vi "AlarmReport.vi"(5 "PalletError":i32, 6 "RooCauseIn":string, 7 "Emun":T1=enum."WriteOPID", 8 "VILinkerror In":errorcluster, 9 "OPID":string, 10 "error In":errorcluster, 11 "ErrorTableIn":refnum<vi>) -> (0 "error out":errorcluster)   [LabVIEW 2019]
uses:
  Ctrl/AlarmReportCtrl.ctl
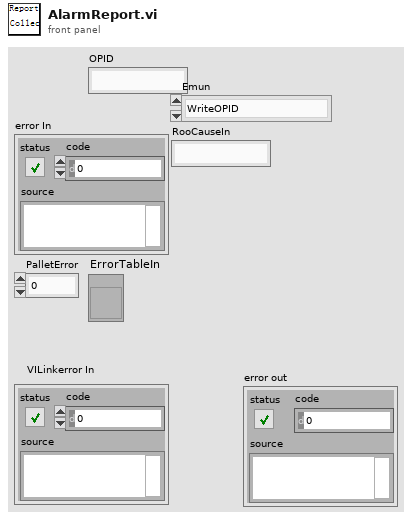
[diagram p1: front panel]
types:
  T1 = typedef "AlarmReportCtrl.ctl" = enum16{"Initial", "AddError", "WriteAlarmResetTime", "WriteOPID", "Load", "Save", "WriteRootCause"}
  T2 = enum16{"open", "replace", "create", "open or create", "replace or create", "replace or create with confirmation"}
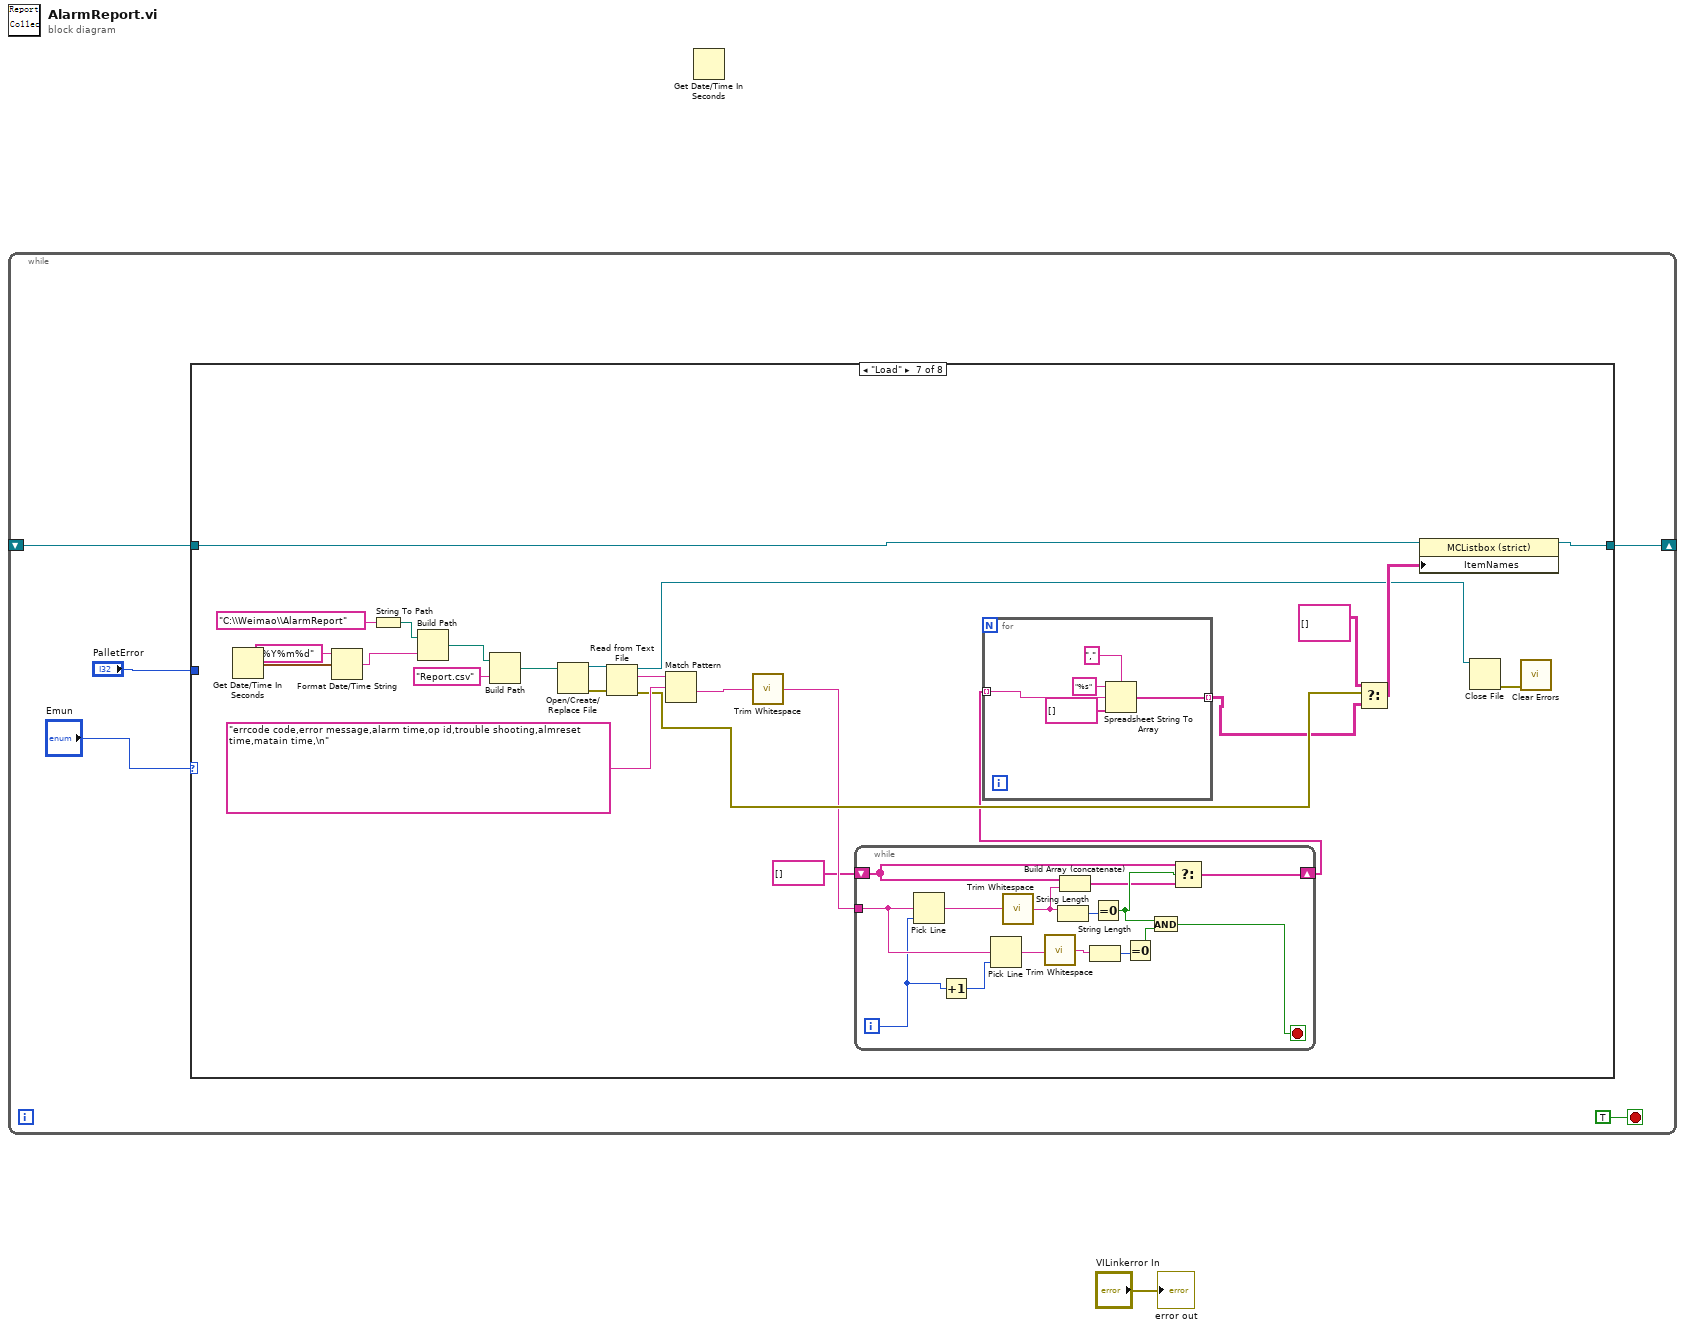
[diagram p0: block diagram]
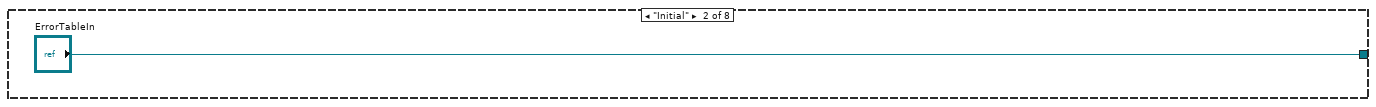
[diagram p3: hidden frame]
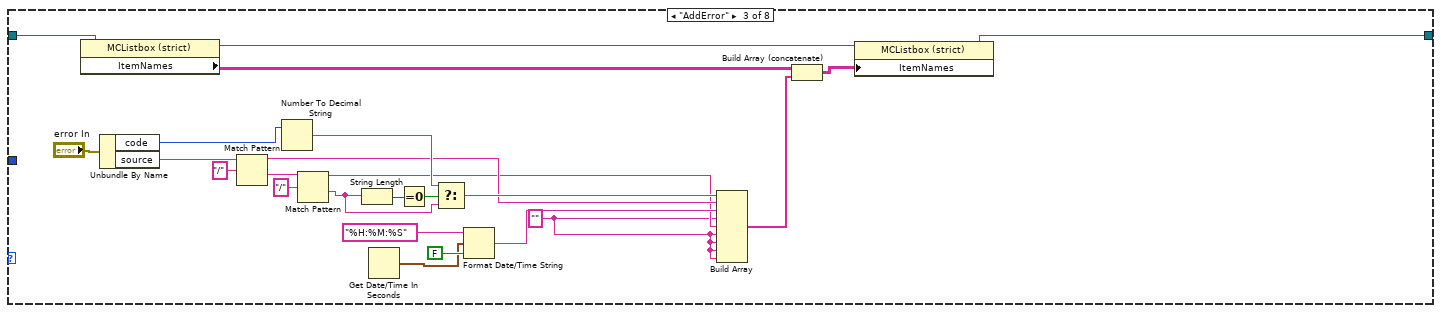
[diagram p4: hidden frame]
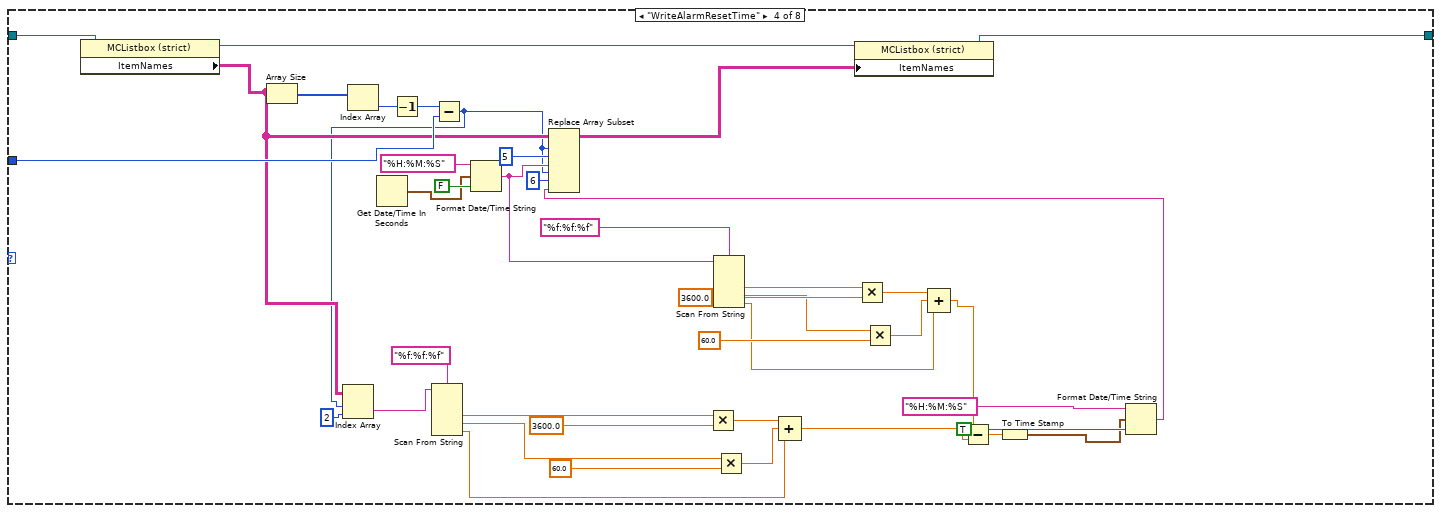
[diagram p5: hidden frame]
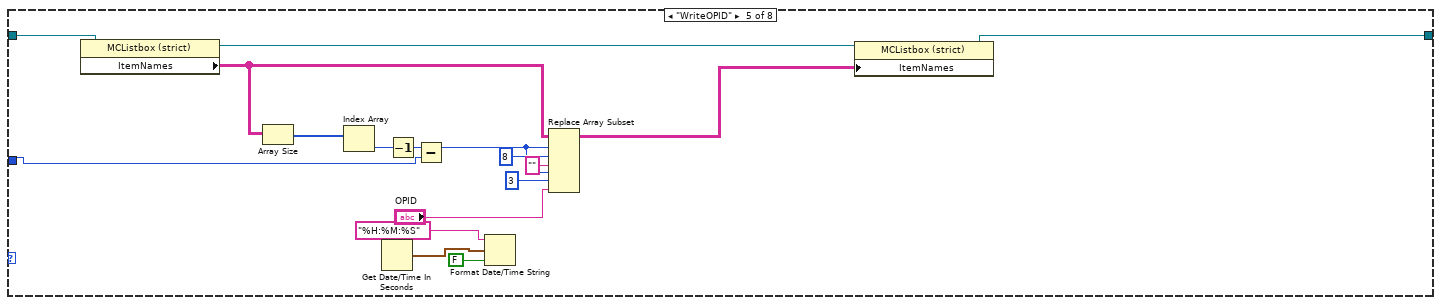
[diagram p6: hidden frame]
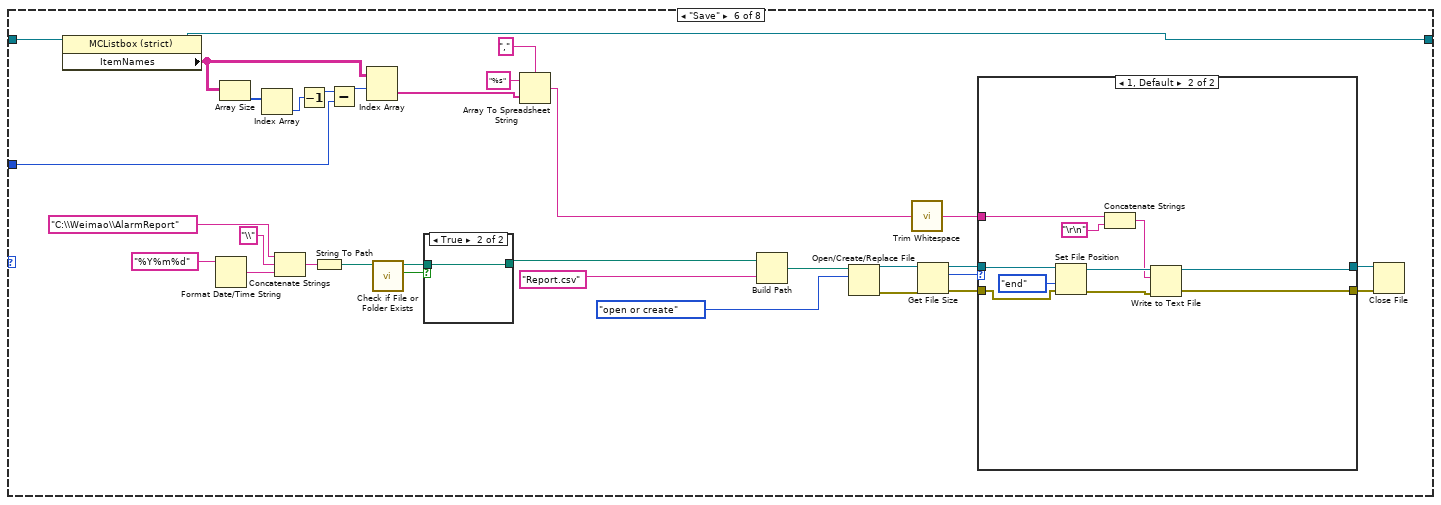
[diagram p7: hidden frame]
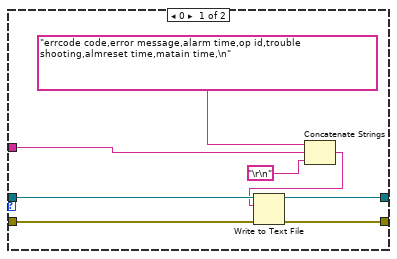
[diagram p8: hidden frame]
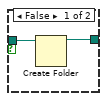
[diagram p9: hidden frame]
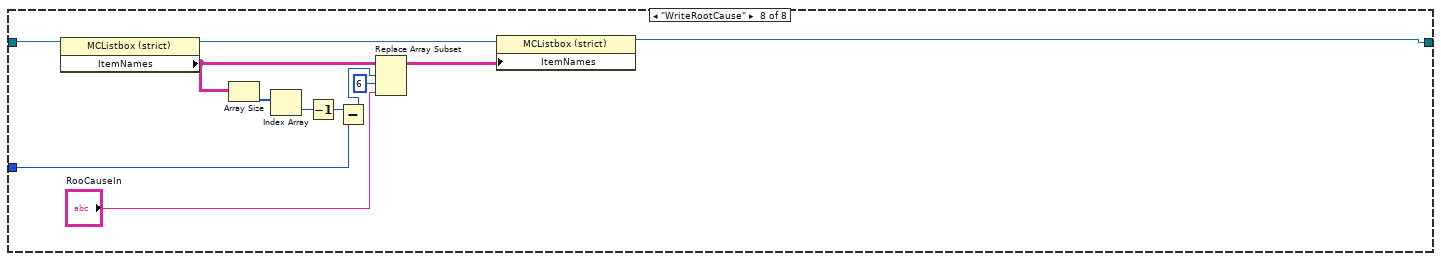
[diagram p10: hidden frame]
diagram:
  n1 = while {
    shift-right: [w4] -> _
    shift-left: _ -> [w3]
    stop <- TRUE stop-if-true
    n2 = case shown="\"Load\"" "Emun" {
      tunnel: [w7 "ErrorTableIn" w12 w71 w88 w121 w166 w191] -> w4
      tunnel: w3 -> [w7 _ w32 w73 w90 w122 w167 w199]
      tunnel: "PalletError" -> [_ _ _ w61 w76 w91 _ w188]
      frame Default {
      }
      frame "Initial" {
      }
      frame "AddError" {
        w15 = "" ("element")
        n3 = property class="MCListbox (strict)"(reference=w32) -> (reference out=w14:refnum<vi>, "ItemNames"=w30:string[][])  [unwired: 1 in, 1 out]
        n4 = Unbundle By Name("error In") -> ("code"=w23:i32, "source"=w29:string)
        n5 = Match Pattern(string=w29, regular expression="/") -> (before substring=w19:string, after substring=w27:string)  [unwired: 1 in, 2 out]
        n6 = Number To Decimal String(number=w23) -> (decimal integer string=w22:string)  [unwired: 1 in]
        n7 = Match Pattern(string=w27, regular expression="/") -> (before substring=w16:string, after substring=w21:string)  [unwired: 1 in, 2 out]
        n8 = String Length(string=w21) -> (length=w25:i32)
        n9 = Get Date/Time In Seconds() -> (seconds since 1Jan1904=w10:timestamp)
        n10 = Equal To 0?(x=w25) -> (x = 0?=w24:bool)
        n11 = Select(t=w22, s=w24, f=w21) -> (s? t:f=w20:string)
        n12 = Format Date/Time String(time format string (%c)="%H:%M:%S", seconds (now)=w10, UTC format=FALSE) -> (date/time string=w17:string)
        n13 = Build Array(w20, w19, w17, w15, w16, w15, w15, w15, w15) -> (w9:string[])
        n14 = Build Array (concatenate)(w30, w9) -> (w13:string[][])
        n15 = property class="MCListbox (strict)"(reference=w14, "ItemNames"=w13) -> (reference out=w12:refnum<vi>)  [unwired: 1 in, 1 out]
      }
      frame "WriteAlarmResetTime" {
        n16 = property class="MCListbox (strict)"(reference=w73) -> (reference out=w72:refnum<vi>, "ItemNames"=w57:string[][])  [unwired: 1 in, 1 out]
        n17 = Array Size(array=w57) -> (size(s)=w69:i32[])
        n18 = Index Array(array=w69) -> (element=w68:i32)  [unwired: 1 in]
        n19 = Get Date/Time In Seconds() -> (seconds since 1Jan1904=w62:timestamp)
        n20 = Decrement(x=w68) -> (x-1=w65:i32)
        n21 = Subtract(x=w65, y=w61) -> (x-y=w33:i32)
        n22 = Index Array(array=w57, index (row)=w33, index (col)=2 ("disabled index (col)")) -> (element=w41:string)
        n23 = Scan From String(format string="%f:%f:%f", input string=w41) -> (output 1=w43:dbl, output 2=w45:dbl, output 3=w49:dbl)  [unwired: 5 in, 3 out]
        n24 = Format Date/Time String(time format string (%c)="%H:%M:%S", seconds (now)=w62, UTC format=FALSE) -> (date/time string=w59:string)
        n25 = Multiply(x=w43, y=3600.0) -> (x*y=w47:dbl)
        n26 = Scan From String(format string="%f:%f:%f", input string=w59) -> (output 1=w58:dbl, output 2=w54:dbl, output 3=w50:dbl)  [unwired: 5 in, 3 out]
        n27 = Multiply(x=w45, y=60.0) -> (x*y=w48:dbl)
        n28 = Compound Arithmetic op=ADD(w47, w48, w49) -> (w35:dbl)
        n29 = Multiply(x=w58, y=3600.0) -> (x*y=w52:dbl)
        n30 = Multiply(x=w54, y=60.0) -> (x*y=w51:dbl)
        n31 = Compound Arithmetic op=ADD(w52, w51, w50) -> (w34:dbl)
        n32 = Subtract(x=w34, y=w35) -> (x-y=w40:dbl)
        n33 = To Time Stamp(1:w40) -> (0:w37:timestamp)
        n34 = Format Date/Time String(time format string (%c)="%H:%M:%S", seconds (now)=w37, UTC format=TRUE) -> (date/time string=w36:string)
        n35 = Replace Array Subset(array=w57, new element #1=w59, index (row) #1=w33, index (col) #1=5 ("disabled index (col)"), new element #2=w36, index (row) #2=w33, index (col) #2=6 ("disabled index (col)")) -> (w70:string[][])
        n36 = property class="MCListbox (strict)"(reference=w72, "ItemNames"=w70) -> (reference out=w71:refnum<vi>)  [unwired: 1 in, 1 out]
      }
      frame "WriteOPID" {
        n37 = property class="MCListbox (strict)"(reference=w90) -> (reference out=w89:refnum<vi>, "ItemNames"=w83:string[][])  [unwired: 1 in, 1 out]
        n38 = Array Size(array=w83) -> (size(s)=w86:i32[])
        n39 = Index Array(array=w86) -> (element=w85:i32)  [unwired: 1 in]
        n40 = Get Date/Time In Seconds() -> (seconds since 1Jan1904=w78:timestamp)
        n41 = Decrement(x=w85) -> (x-1=w81:i32)
        n42 = Subtract(x=w81, y=w76) -> (x-y=w77:i32)
        n43 = Format Date/Time String(time format string (%c)="%H:%M:%S", seconds (now)=w78, UTC format=FALSE) -> ()  [unwired: 1 out]
        n44 = Replace Array Subset(array=w83, new element #1="" ("new element/subarray"), index (row) #1=w77, index (col) #1=8 ("disabled index (col)"), new element #2="OPID", index (row) #2=w77, index (col) #2=3 ("disabled index (col)")) -> (w87:string[][])
        n45 = property class="MCListbox (strict)"(reference=w89, "ItemNames"=w87) -> (reference out=w88:refnum<vi>)  [unwired: 1 in, 1 out]
      }
      frame "Save" {
        n46 = property class="MCListbox (strict)"(reference=w122) -> (reference out=w121:refnum<vi>, "ItemNames"=w105:string[][])  [unwired: 1 in, 1 out]
        n47 = Format Date/Time String(time format string (%c)="%Y%m%d") -> (date/time string=w118:string)  [unwired: 2 out]
        n48 = Array Size(array=w105) -> (size(s)=w104:i32[])
        n49 = Index Array(array=w104) -> (element=w103:i32)  [unwired: 1 in]
        n50 = Concatenate Strings("C:\\Weimao\\AlarmReport" ("LogFolder"), "\\" ("string"), w118) -> (w117:string)
        n51 = Decrement(x=w103) -> (x-1=w92:i32)
        n52 = String To Path(string=w117) -> (path=w115:path)
        n53 = Subtract(x=w92, y=w91) -> (x-y=w93:i32)
        n54 = Index Array(array=w105, index (row)=w93) -> (element=w102:string[])  [unwired: 1 in]
        n55 = call <vilib>:"Check if File or Folder Exists.vi"("path"=w115) -> ("file or folder exists?"=w113:bool, "dup path"=w114:path)  [unwired: 8 in, 1 out]
        n56 = case shown="True" w113 {
          tunnel: w114 -> [w142 w143]
          tunnel: [w141 w143] -> w112
          frame False {
            n57 = Create Folder(path (use dialog)=w142) -> (created path=w141:path)  [unwired: 2 in, 2 out]
          }
          frame True {
          }
        }
        n58 = Array To Spreadsheet String(delimiter (Tab)=",", array=w102, 3:"%s" ("format string")) -> (spreadsheet string=w99:string)
        n59 = Build Path(base path=w112, name or relative path="Report.csv") -> (appended path=w110:path)
        n60 = Open/Create/Replace File(file path (use dialog)=w110, operation (0:open)=T2."open or create") -> (refnum out=w108:refnum<file>, error out=w107:errorcluster)  [unwired: 4 in, 1 out]
        n61 = call <vilib>:"Trim Whitespace.vi"("string"=w99) -> ("trimmed string"=w94:string)  [unwired: 1 in]
        n62 = Get File Size(file=w108, error in=w107) -> (refnum out=w98:refnum<file>, size (in bytes)=w106:i64, 0:w97:errorcluster)
        n63 = case shown="1, Default" w106 {
          tunnel: w94 -> [w129 w135]
          tunnel: w98 -> [w128 w140]
          tunnel: w97 -> [w127 w138]
          tunnel: [w126 w134] -> w95
          tunnel: [w125 w133] -> w96
          frame 0 {
            n64 = Concatenate Strings("errcode code,error message,alarm time,op id,trouble shooting,almreset time,matain time,\n", w129, "\r\n") -> (w123:string)
            n65 = Write to Text File(file (use dialog)=w128, text=w123, error in=w127) -> (refnum out=w126:refnum<file>, error out=w125:errorcluster)  [unwired: 1 in, 1 out]
          }
          frame 1, Default {
            n66 = Set File Position(refnum=w140, from (0:start)=enum16{"start", "end", "current"}."end", error in=w138) -> (refnum out=w137:refnum<file>, error out=w136:errorcluster)  [unwired: 1 in]
            n67 = Concatenate Strings(w135, "\r\n") -> (w132:string)
            n68 = Write to Text File(file (use dialog)=w137, text=w132, error in=w136) -> (refnum out=w134:refnum<file>, error out=w133:errorcluster)  [unwired: 1 in, 1 out]
          }
        }
        n69 = Close File(refnum=w95, error in=w96) -> ()  [unwired: 2 out]
      }
      frame "Load" {
        n70 = Get Date/Time In Seconds() -> (seconds since 1Jan1904=w165:timestamp)
        n71 = Format Date/Time String(time format string (%c)="%Y%m%d", seconds (now)=w165) -> (date/time string=w161:string)  [unwired: 1 in]
        n72 = String To Path(string="C:\\Weimao\\AlarmReport" ("LogFolder")) -> (path=w162:path)
        n73 = Build Path(base path=w162, name or relative path=w161) -> (appended path=w160:path)
        n74 = Build Path(base path=w160, name or relative path="Report.csv") -> (appended path=w158:path)
        n75 = Open/Create/Replace File(file path (use dialog)=w158) -> (refnum out=w157:refnum<file>, error out=w156:errorcluster)  [unwired: 5 in, 1 out]
        n76 = Read from Text File(file (use dialog)=w157, error in=w156) -> (refnum out=w147:refnum<file>, text=w153:string, error out=w150:errorcluster)  [unwired: 2 in, 1 out]
        n77 = Match Pattern(string=w153, regular expression="errcode code,error message,alarm time,op id,trouble shooting,almreset time,matain time,\n") -> (after substring=w151:string)  [unwired: 1 in, 3 out]
        n78 = call <vilib>:"Trim Whitespace.vi"("string"=w151) -> ("trimmed string"=w148:string)  [unwired: 1 in]
        n79 = while {
          tunnel: w148 -> [w181]
          shift-right: [w171] -> w145
          shift-left: string[] [] -> [w168]
          i -> [w180]
          stop <- w173 stop-if-true
          n80 = Pick Line(multi-line string=w181, line index=w180) -> (output string=w179:string)  [unwired: 1 in]
          n81 = Increment(x=w180) -> (x+1=w182:i32)
          n82 = Pick Line(multi-line string=w181, line index=w182) -> (output string=w178:string)  [unwired: 1 in]
          n83 = call <vilib>:"Trim Whitespace.vi"("string"=w179) -> ("trimmed string"=w169:string)  [unwired: 1 in]
          n84 = call <vilib>:"Trim Whitespace.vi"("string"=w178) -> ("trimmed string"=w175:string)  [unwired: 1 in]
          n85 = String Length(string=w169) -> (length=w177:i32)
          n86 = Build Array (concatenate)(w168, w169) -> (w170:string[])
          n87 = String Length(string=w175) -> (length=w176:i32)
          n88 = Equal To 0?(x=w177) -> (x = 0?=w172:bool)
          n89 = Equal To 0?(x=w176) -> (x = 0?=w174:bool)
          n90 = And(x=w172, y=w174) -> (x .and. y?=w173:bool)
          n91 = Select(t=w168, s=w172, f=w170) -> (s? t:f=w171:string[])
        }
        n92 = for {
          tunnel: w145 -> [w185] mode=indexing
          tunnel: [w183] -> w144 mode=indexing
          n93 = Spreadsheet String To Array(delimiter (Tab)=",", format string="%s", spreadsheet string=w185, array type (2D Dbl)=string[] []) -> (array=w183:string[])
        }
        n94 = Select(t=string[][] [] ("Value"), s=w150, f=w144) -> (s? t:f=w154:string[][])
        n95 = property class="MCListbox (strict)"(reference=w167, "ItemNames"=w154) -> (reference out=w166:refnum<vi>)  [unwired: 1 in, 1 out]
        n96 = Close File(refnum=w147) -> (error out=w149:errorcluster)  [unwired: 1 in, 1 out]
        n97 = call <vilib>:"Clear Errors.vi"("error in (no error)"=w149) -> ()  [unwired: 5 in, 2 out]
      }
      frame "WriteRootCause" {
        n98 = property class="MCListbox (strict)"(reference=w199) -> (reference out=w194:refnum<vi>, "ItemNames"=w196:string[][])  [unwired: 1 in, 1 out]
        n99 = Array Size(array=w196) -> (size(s)=w198:i32[])
        n100 = Index Array(array=w198) -> (element=w197:i32)  [unwired: 1 in]
        n101 = Decrement(x=w197) -> (x-1=w190:i32)
        n102 = Subtract(x=w190, y=w188) -> (x-y=w189:i32)
        n103 = Replace Array Subset(array=w196, new element="RooCauseIn", index (row)=w189, index (col)=6 ("disabled index (col)")) -> (w193:string[][])
        n104 = property class="MCListbox (strict)"(reference=w194, "ItemNames"=w193) -> (reference out=w191:refnum<vi>)  [unwired: 1 in, 1 out]
      }
    }
  }
  n105 = Get Date/Time In Seconds() -> ()  [unwired: 1 out]
  "error out" <- "VILinkerror In"
